vi "update.vi"(8 "error in (no error)":errorcluster, 10 "adapter executability":T1={"instrument"=TRUE, "trajectory"=TRUE, "scanHead"=TRUE, "DAQ"=TRUE, "imageAssembler"=TRUE, "dataCollection"=TRUE, "display"=TRUE, "analyser"=TRUE, "stimulator"=TRUE}, 11 "ImagingModeDL090130Frame in":refnum<class "ImagingModeDL090130Frame.lvclass">=refnum) -> (0 "error out":errorcluster, 3 "ImagingModeDL090130Frame out":refnum<class "ImagingModeDL090130Frame.lvclass">)   [LabVIEW 2010, in "ImagingModeDL090130Frame.lvclass"]
uses:
  ImagingModeDL090130Frame.lvclass
  ImagingModeDL090923Scaffold/ImagingModeDL090923Scaffold/adapter_executability_cluster.ctl
  ImagingModeDL090923Scaffold/ImagingModeDL090923Scaffold/ImagingModeDL090923Scaffold.lvclass
  ScanHead/GenericScanHead/GenericScanHead/GenericScanHead.lvclass
  ImageAssembler/GenericImageAssembler/GenericImageAssembler/GenericImageAssembler.lvclass
  DataCollection/GenericDataCollection/GenericDataCollection/GenericDataCollection.lvclass
  common/xcontrols/XSettings/XSettings/XSettings.xctl
  common/classes/ErrorController/ErrorController/class_data.vi
  common/classes/ErrorController/ErrorController/ErrorController.lvclass
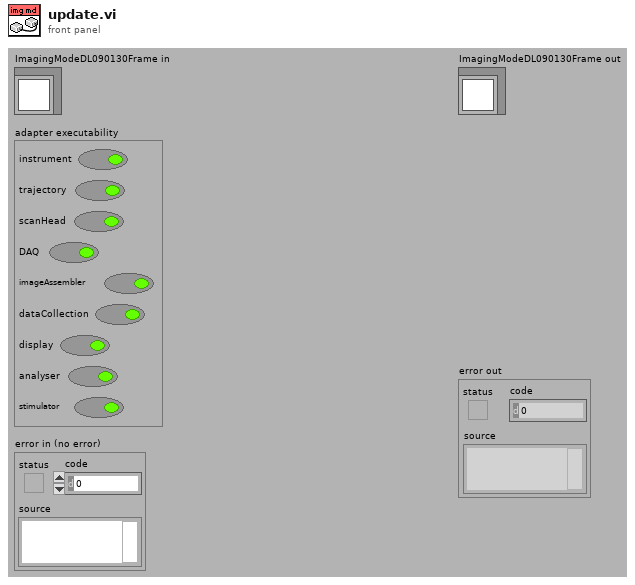
[diagram p1: front panel]
types:
  T1 = typedef "ImagingModeDL090923Scaffold.lvclass/adapter_executability_cluster.ctl" = cluster{"instrument":bool, "trajectory":bool, "scanHead":bool, "DAQ":bool, "imageAssembler":bool, "dataCollection":bool, "display":bool, "analyser":bool, "stimulator":bool}
  T2 = typedef "ImagingModeDL090130Frame.lvclass/control_refs.ctl" = cluster{"resolution controls":cluster{"x pixels":refnum<vi>, "y pixels":refnum<vi>, "ratio x factor":refnum<vi>, "ratio y factor":refnum<vi>}, "speed controls":cluster{"pixel dwell time":refnum<vi>, "line scan time":refnum<vi>, "frame rate":refnum<vi>, "keep constant":refnum<vi>}, "number of frames controls":cluster{"# of frames":refnum<vi>, "duration":refnum<vi>, "# of repetitions":refnum<vi>}, "current value indicators":cluster{"frame #":refnum<vi>, "repetition #":refnum<vi>, "offset":refnum<vi>}, "step controls":cluster{"step size":refnum<vi>, "return to origin?":refnum<vi>, "translation mode":refnum<vi>, "XIntensityCompensation":refnum<vi>}, "defineButton":refnum<vi>, "settings enforced?":refnum<vi>, "settings":refnum<vi>}
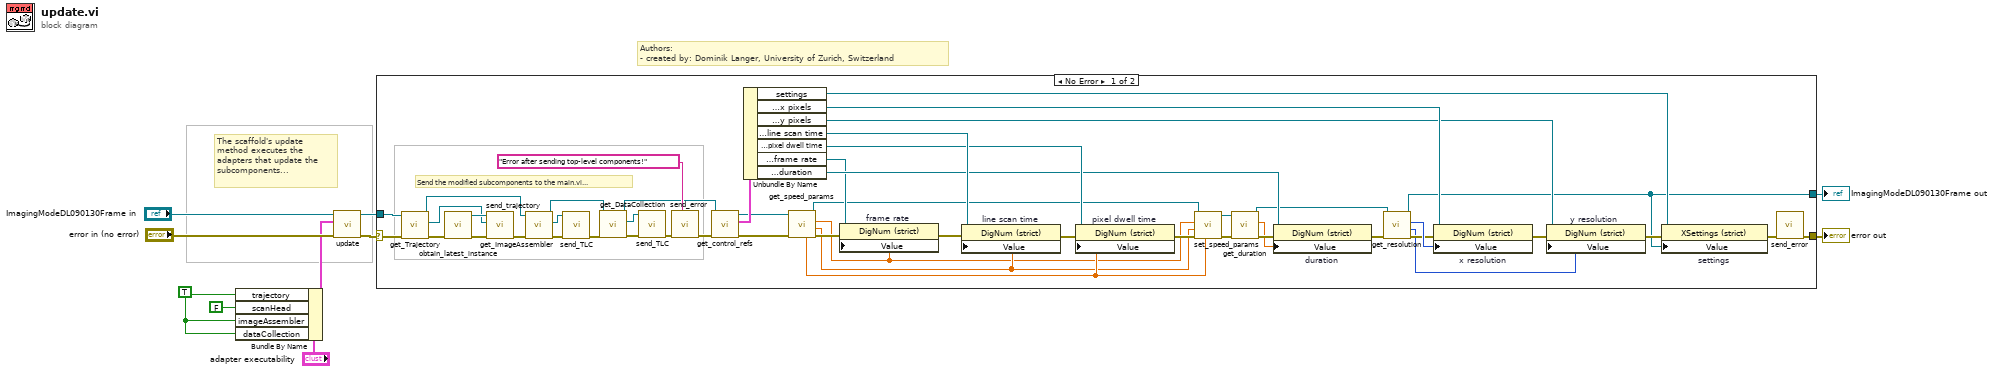
[diagram p0: block diagram]
diagram:
  w2 = TRUE ("instrument")
  # "The scaffold's update method executes the adapters that update the subcomponents..."
  # "Authors: \n- created by: Dominik Langer, University of Zurich, Switzerland"
  n1 = Bundle By Name(cluster="adapter executability", "trajectory"=w2, "scanHead"=FALSE ("instrument"), "imageAssembler"=w2, "dataCollection"=w2) -> (w1:T1)
  n2 = call-parent "update.vi"("error in (no error)"="error in (no error)", "adapter executability"=w1, "ScanModeDL090923Scaffold in"="ImagingModeDL090130Frame in") -> ("error out"=w6:errorcluster, "ScanModeDL090923Scaffold out"=w5:refnum<class "ImagingModeDL090130Frame.lvclass">)  [unwired: 7 in]
  n3 = case shown="No Error" w6 {
    selector: w6 -> [w57 w62]
    tunnel: [w39 w62] -> w10
    tunnel: [w11 w61] -> w9
    tunnel: w5 -> [w56 w61]
    frame No Error {
      # "Send the modified subcomponents to the main.vi..."
      n4 = call-dynamic "get_Trajectory.vi"("error in (no error)"=w57, "ScanModeDL090923Scaffold in"=w56) -> ("error out"=w44:errorcluster, "Trajectory"=w42:refnum<class "GenericTrajectory.lvclass">, "ScanModeDL090923Scaffold out"=w43:refnum<class "ImagingModeDL090130Frame.lvclass">)  [unwired: 2 in, 5 out]
      n5 = call "obtain_latest_instance.vi"("error in (no error)"=w44) -> ("error out"=w45:errorcluster, "GenericScanHead out"=w47:refnum<class "GenericScanHead.lvclass">)  [unwired: 1 in, 8 out]
      n6 = call-dynamic "send_trajectory.vi"("error in (no error)"=w45, "trajectory"=w42, "GenericScanHead in"=w47) -> ("error out"=w46:errorcluster)  [unwired: 8 out]
      n7 = call-dynamic "get_ImageAssembler.vi"("error in (no error)"=w46, "ScanModeDL090923Scaffold in"=w43) -> ("error out"=w55:errorcluster, "ImageAssembler"=w54:refnum<class "GenericImageAssembler.lvclass">, "ScanModeDL090923Scaffold out"=w50:refnum<class "ImagingModeDL090130Frame.lvclass">)  [unwired: 4 in, 3 out]
      n8 = call-dynamic "send_TLC.vi"("error in (no error)"=w55, "GenericToplevelComponent in"=w54) -> ("error out"=w52:errorcluster)  [unwired: 8 in, 1 out]
      n9 = call-dynamic "get_DataCollection.vi"("error in (no error)"=w52, "ScanModeDL090923Scaffold in"=w50) -> ("error out"=w53:errorcluster, "DataCollection"=w51:refnum<class "GenericDataCollection.lvclass">, "ScanModeDL090923Scaffold out"=w26:refnum<class "ImagingModeDL090130Frame.lvclass">)  [unwired: 4 in, 3 out]
      n10 = call-dynamic "send_TLC.vi"("error in (no error)"=w53, "GenericToplevelComponent in"=w51) -> ("error out"=w40:errorcluster)  [unwired: 8 in, 1 out]
      n11 = call "send_error.vi"("additional message"="Error after sending top-level components!", "error in (no error)"=w40) -> ("error out"=w29:errorcluster)  [unwired: 9 in]
      n12 = call-dynamic "get_control_refs.vi"("error in (no error)"=w29, "ImagingModeDL090130Frame in"=w26) -> ("error out"=w28:errorcluster, "control refs"=w27:T2, "ImagingModeDL090130Frame out"=w25:refnum<class "ImagingModeDL090130Frame.lvclass">)  [unwired: 7 in]
      n13 = Unbundle By Name(w27) -> ("settings"=w14:refnum<vi>, "resolution controls.x pixels"=w23:refnum<vi>, "resolution controls.y pixels"=w22:refnum<vi>, "speed controls.line scan time"=w60:refnum<vi>, "speed controls.pixel dwell time"=w59:refnum<vi>, "speed controls.frame rate"=w37:refnum<vi>, "number of frames controls.duration"=w58:refnum<vi>)
      n14 = call-dynamic "get_speed_params.vi"("error in (no error)"=w28, "ImagingModeDL090130Frame in"=w25) -> ("error out"=w36:errorcluster, "line-scan time"=w16:dbl[unit], "frame rate"=w15:dbl[unit], "ImagingModeDL090130Frame out"=w21:refnum<class "ImagingModeDL090130Frame.lvclass">, "pixel dwell time"=w17:dbl[unit])  [unwired: 4 in, 1 out]
      n15 = property on="frame rate" class="DigNum (strict)"(reference=w37, error in=w36, "Value"=w15) -> (error out=w35:errorcluster)  [unwired: 1 out]
      n16 = property on="line scan time" class="DigNum (strict)"(reference=w60, error in=w35, "Value"=w16) -> (error out=w41:errorcluster)  [unwired: 1 out]
      n17 = property on="pixel dwell time" class="DigNum (strict)"(reference=w59, error in=w41, "Value"=w17) -> (error out=w19:errorcluster)  [unwired: 1 out]
      n18 = call-dynamic "set_speed_params.vi"("pixel-dwell time"=w17, "error in (no error)"=w19, "line-scan time"=w16, "frame rate"=w15, "ImagingModeDL090130Frame in"=w21) -> ("error out"=w18:errorcluster, "ImagingModeDL090130Frame out"=w20:refnum<class "ImagingModeDL090130Frame.lvclass">)  [unwired: 5 in]
      n19 = call-dynamic "get_duration.vi"("error in (no error)"=w18, "ImagingModeDL090130Frame in"=w20) -> ("error out"=w49:errorcluster, "duration"=w48:dbl[unit], "ImagingModeDL090130Frame out"=w24:refnum<class "ImagingModeDL090130Frame.lvclass">)  [unwired: 7 out]
      n20 = property on="duration" class="DigNum (strict)"(reference=w58, error in=w49, "Value"=w48) -> (error out=w34:errorcluster)  [unwired: 1 out]
      n21 = call-dynamic "get_resolution.vi"("error in (no error)"=w34, "ImagingModeDL090130Frame in"=w24) -> ("error out"=w32:errorcluster, "y resolution"=w30:i32, "x resolution"=w33:i32, "ImagingModeDL090130Frame out"=w11:refnum<class "ImagingModeDL090130Frame.lvclass">)  [unwired: 6 in]
      n22 = property on="x resolution" class="DigNum (strict)"(reference=w23, error in=w32, "Value"=w33) -> (error out=w31:errorcluster)  [unwired: 1 out]
      n23 = property on="y resolution" class="DigNum (strict)"(reference=w22, error in=w31, "Value"=w30) -> (error out=w13:errorcluster)  [unwired: 1 out]
      n24 = property on="settings" class="XSettings (strict)"(reference=w14, error in=w13, "Value"=w11) -> (error out=w12:errorcluster)  [unwired: 1 out]
      n25 = call "send_error.vi"("error in (no error)"=w12) -> ("error out"=w39:errorcluster)  [unwired: 10 in]
    }
    frame Error {
    }
  }
  "error out" <- w10
  "ImagingModeDL090130Frame out" <- w9
